vi "Toolkit Post-Install Custom Action.vi"(10 "Variant":variant) -> (0 "error out":errorcluster)   [LabVIEW 2020]
uses:
  <vilib>/Utility/traverseref.llb/TRef TravTarget.ctl
  <vilib>/Utility/traverseref.llb/VI Scripting - Traverse.lvlib
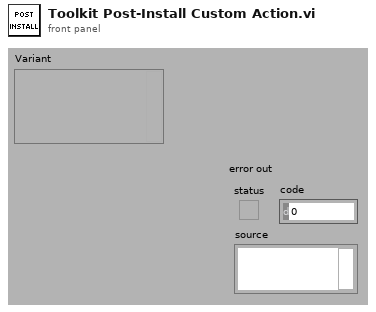
[diagram p1: front panel]
types:
  T1 = typedef "TRef TravTarget.ctl" = enum16{"FP", "BD", "Other"}
  T2 = typedef "LVPositionTypeDef.ctl" = cluster{"Left":i32, "Top":i32}
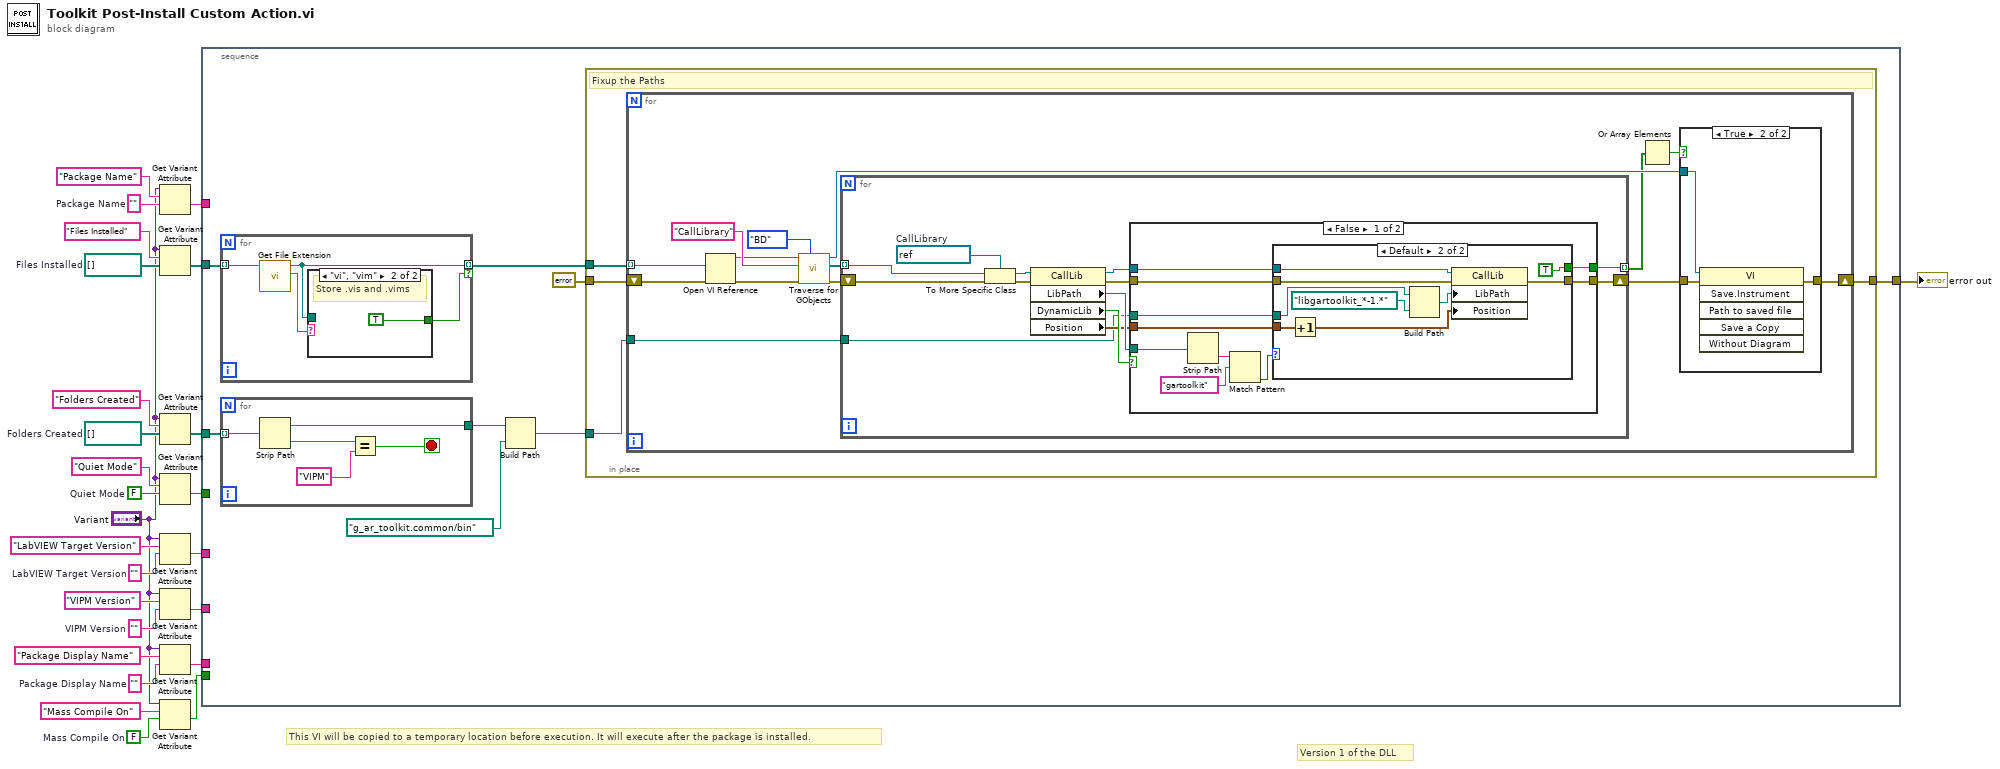
[diagram p0: block diagram]
diagram:
  w3 = path[] []  # Folders Created
  w4 = path[] []  # Files Installed
  w9 = FALSE  # Mass Compile On
  w10 = ""  # Package Display Name
  w17 = FALSE  # Quiet Mode
  w20 = ""  # VIPM Version
  w22 = ""  # LabVIEW Target Version
  w24 = ""  # Package Name
  # "Version 1 of the DLL"
  # "This VI will be copied to a temporary location before execution. It will execute after the package is installed."
  n1 = Get Variant Attribute(Variant="Variant", name="Package Name", default value (empty Variant)=w24) -> (value=w15:string)  [unwired: 1 in, 3 out]
  n2 = Get Variant Attribute(Variant="Variant", name="Files Installed", default value (empty Variant)=w4) -> (value=w6:path[])  [unwired: 1 in, 3 out]
  n3 = Get Variant Attribute(Variant="Variant", name="Folders Created", default value (empty Variant)=w3) -> (value=w7:path[])  [unwired: 1 in, 3 out]
  n4 = Get Variant Attribute(Variant="Variant", name="Quiet Mode", default value (empty Variant)=w17) -> (value=w12:bool)  [unwired: 1 in, 3 out]
  n5 = Get Variant Attribute(Variant="Variant", name="LabVIEW Target Version", default value (empty Variant)=w22) -> (value=w14:string)  [unwired: 1 in, 3 out]
  n6 = Get Variant Attribute(Variant="Variant", name="VIPM Version", default value (empty Variant)=w20) -> (value=w13:string)  [unwired: 1 in, 3 out]
  n7 = Get Variant Attribute(Variant="Variant", name="Package Display Name", default value (empty Variant)=w10) -> (value=w16:string)  [unwired: 1 in, 3 out]
  n8 = Get Variant Attribute(Variant="Variant", name="Mass Compile On", default value (empty Variant)=w9) -> (value=w11:bool)  [unwired: 1 in, 3 out]
  n9 = stacked-sequence {
    tunnel: w16 -> [_]
    tunnel: w15 -> [_]
    tunnel: w14 -> [_]
    tunnel: w13 -> [_]
    tunnel: w12 -> [_]
    tunnel: w11 -> [_]
    tunnel: w6 -> [w34]
    tunnel: w7 -> [w33]
    tunnel: [w29] -> w2
    frame #0 {
      n10 = for {
        tunnel: w34 -> [w43] mode=indexing
        tunnel: [w40] -> w32 mode=indexing if=w41
        n11 = call <vilib>:"Get File Extension.vi"("file"=w43) -> ("lowercase file extension"=w42:string, "dup file"=w40:path)  [unwired: 6 in, 3 out]
        n12 = case shown="\"vi\", \"vim\"" w42 {
          tunnel: [_ TRUE] -> w41
          tunnel: w40 -> [_ _]
          frame Default {
          }
          frame "vi", "vim" {
            # "Store .vis and .vims"
          }
        }
      }
      n13 = for {
        tunnel: w33 -> [w39] mode=indexing
        tunnel: [w38] -> w28
        stop <- w36 stop-if-true
        n14 = Strip Path(path=w39) -> (stripped path=w38:path, name=w37:string)
        n15 = Equal?(x=w37, y="VIPM") -> (x = y?=w36:bool)
      }
      n16 = Build Path(base path=w28, name or relative path=path "g_ar_toolkit.common/bin") -> (appended path=w30:path)
      n17 = in-place {
        in-place-border: [w46] -> w29
        in-place-border: w32 -> [w48]
        in-place-border: errorcluster {"status"=FALSE, "code"=0, "source"=""} ("error in (no error)") -> [w47]
        in-place-border: w30 -> [w45]
        # "Fixup the Paths"
        n18 = for {
          tunnel: w48 -> [w60] mode=indexing
          shift-right: [w58] -> w46
          shift-left: w47 -> [w57]
          tunnel: w45 -> [w49]
          n19 = Open VI Reference(vi path=w60, error in (no error)=w57) -> (vi reference=w53:refnum<vi>, error out=w52:errorcluster)  [unwired: 4 in]
          n20 = call <vilib>:"Traverse for GObjects.vi"("Traverse Target"=TRef_TravTarget."BD", "error in (no error)"=w52, "Class Name"="CallLibrary", "VI Refnum"=w53) -> ("error out"=w56:errorcluster, "References"=w51:refnum<vi>[], "dup VI Refnum"=w62:refnum<vi>)  [unwired: 4 in, 1 out]
          n21 = for {
            tunnel: w51 -> [w68] mode=indexing
            shift-right: [w75] -> w61
            shift-left: w56 -> [w70]
            tunnel: [w66] -> w50 mode=indexing
            tunnel: w49 -> [w63]
            w69 = refnum<vi> refnum  # CallLibrary
            n22 = To More Specific Class(target class=w69, reference=w68, error in=w70) -> (specific class reference=w71:refnum<vi>, error out=w72:errorcluster)
            n23 = property class="CallLib"(reference=w71, error in=w72) -> (reference out=w74:refnum<vi>, error out=w73:errorcluster, "LibPath"=w65:path, "DynamicLib"=w67:bool, "Position"=w64:T2)
            n24 = case shown="False" w67 {
              tunnel: [w85 w96] -> w75
              tunnel: w74 -> [w84 _]
              tunnel: w73 -> [w83 w96]
              tunnel: w65 -> [w80 _]
              tunnel: [w79 _] -> w66
              tunnel: w64 -> [w77 _]
              tunnel: w63 -> [w76 _]
              frame False {
                n25 = Strip Path(path=w80) -> (name=w81:string)  [unwired: 1 out]
                n26 = Match Pattern(string=w81, regular expression="gartoolkit") -> (offset past match=w78:i32)  [unwired: 1 in, 3 out]
                n27 = case shown="Default" w78 {
                  tunnel: [w86 w95] -> w85
                  tunnel: w84 -> [_ w93]
                  tunnel: w83 -> [w86 w92]
                  tunnel: [_ TRUE] -> w79
                  tunnel: w77 -> [_ w89]
                  tunnel: w76 -> [_ w87]
                  frame -1 {
                  }
                  frame Default {
                    n28 = Increment(x=w89) -> (x+1=w90:T2)
                    n29 = Build Path(base path=w87, name or relative path=path "libgartoolkit_*-1.*") -> (appended path=w94:path)
                    n30 = property class="CallLib"(reference=w93, error in=w92, "LibPath"=w94, "Position"=w90) -> (error out=w95:errorcluster)  [unwired: 1 out]
                  }
                }
              }
              frame True {
              }
            }
          }
          n31 = Or Array Elements(Boolean array=w50) -> (logical OR=w59:bool)
          n32 = case shown="True" w59 {
            tunnel: w62 -> [_ w99]
            tunnel: w61 -> [w97 w98]
            tunnel: [w97 w100] -> w58
            frame False {
            }
            frame True {
              n33 = invoke class="VI" method="Save.Instrument"(reference=w99, error in=w98) -> (error out=w100:errorcluster)  [unwired: 4 in, 5 out]
            }
          }
        }
      }
    }
  }
  "error out" <- w2
